vi "Disable Source Separation (Project Item).vi"(8 "Error In":errorcluster, 11 "Project Item":refnum<vi>) -> (0 "Error Out":errorcluster, 3 "Project Item Dup":refnum<vi>)   [LabVIEW 2014]
doc: "Copyright (c) 2018 Sze Howe Koh\n\nThis Source Code Form is subject to the terms of the Mozilla Public License, v. 2.0. If a copy of the MPL was not distributed with this file, You can obtain one at http://mozilla.org/MPL/2.0/."
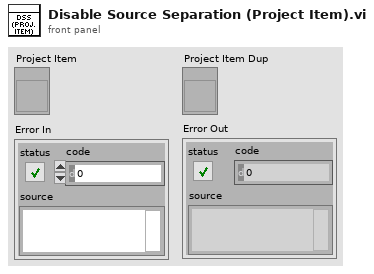
[diagram p1: front panel]
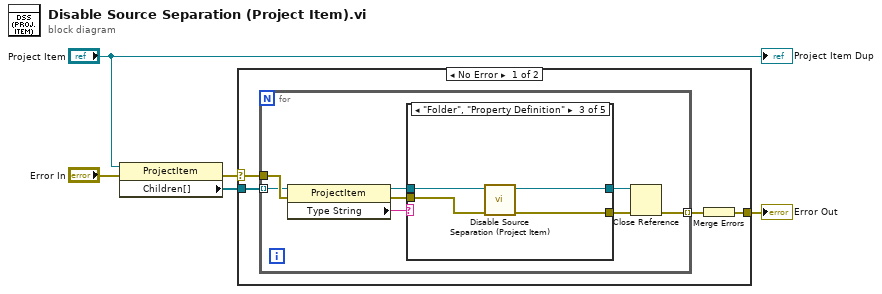
[diagram p0: block diagram]
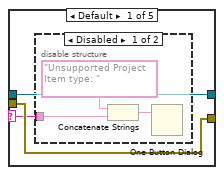
[diagram p2: hidden frame]
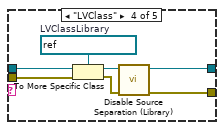
[diagram p5: hidden frame]
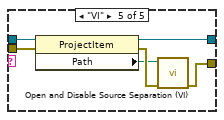
[diagram p6: hidden frame]
diagram:
  n1 = property class="ProjectItem"(reference="Project Item", error in="Error In") -> (error out=w1:errorcluster, "Children[]"=w5:refnum<vi>[])  [unwired: 1 out]
  n2 = case shown="No Error" w1 {
    selector: w1 -> [w9 w43]
    tunnel: w5 -> [w8 _]
    tunnel: [w6 w43] -> w3
    frame No Error {
      n3 = for {
        tunnel: w8 -> [w16] mode=indexing
        tunnel: w9 -> [w17]
        tunnel: [w10] -> w7 mode=indexing
        n4 = property class="ProjectItem"(reference=w16, error in=w17) -> (reference out=w14:refnum<vi>, error out=w12:errorcluster, "Type String"=w15:string)
        n5 = case shown="\"Folder\", \"Property Definition\"" w15 {
          selector: w15 -> [w18 _ _ _ _]
          tunnel: w14 -> [w19 w25 w29 w36 w41]
          tunnel: [w19 w25 w28 w33 w39] -> w13
          tunnel: w12 -> [w20 w24 w27 w32 w38]
          tunnel: [w20 w24 w26 w30 w37] -> w11
          frame Default {
            n6 = disable-structure shown="Disabled" {
              disable-tunnel: w18 -> [w23 _]
              frame Disabled {
                n7 = Concatenate Strings("Unsupported Project Item type: " ("string"), w23) -> (w21:string)
                n8 = One Button Dialog(message=w21) -> ()  [unwired: 1 in, 1 out]
              }
              frame Enabled {
                # "#TODO: Report to caller"
              }
            }
          }
          frame "Class Private Data" {
          }
          frame "Folder", "Property Definition" {
            n9 = call "Disable Source Separation (Project Item).vi"("Error In"=w27, "Project Item"=w29) -> ("Error Out"=w26:errorcluster, "Project Item Dup"=w28:refnum<vi>)  [unwired: 8 in]
          }
          frame "LVClass" {
            w35 = refnum<vi> refnum  # LVClassLibrary
            n10 = To More Specific Class(target class=w35, reference=w36, error in=w32) -> (specific class reference=w34:refnum<vi>, error out=w31:errorcluster)
            n11 = call "Disable Source Separation (Library).vi"("Error In"=w31, "Library"=w34) -> ("Error Out"=w30:errorcluster, "Modded Library"=w33:refnum<vi>)  [unwired: 8 in]
          }
          frame "VI" {
            n12 = property class="ProjectItem"(reference=w41, error in=w38) -> (reference out=w39:refnum<vi>, error out=w42:errorcluster, "Path"=w40:path)
            n13 = call "Open and Disable Source Separation (VI).vi"("Error In"=w42, "VI Path"=w40) -> ("Error Out"=w37:errorcluster)  [unwired: 9 in]
          }
        }
        n14 = Close Reference(reference=w13, error in (no error)=w11) -> (error out=w10:errorcluster)
      }
      n15 = Merge Errors(w7) -> (w6:errorcluster)
    }
    frame Error {
    }
  }
  "Error Out" <- w3
  "Project Item Dup" <- "Project Item"
